vi "Readable.vi"(8 "error in (no error)":errorcluster, 9 "Channel Units":T1, 10 "Channel Names":T2, 11 "Readable in":refnum<class "Readable.lvclass">) -> (0 "error out":errorcluster, 3 "Readable out":refnum<class "Readable.lvclass">)   [LabVIEW 2017, in "Readable.lvclass"]
uses:
  Readable.lvclass
  Channel Names.ctl
  Channel Units.ctl
  Data Point.ctl
  Time.ctl
  X.ctl
  Readable.lvclass/Readable.ctl
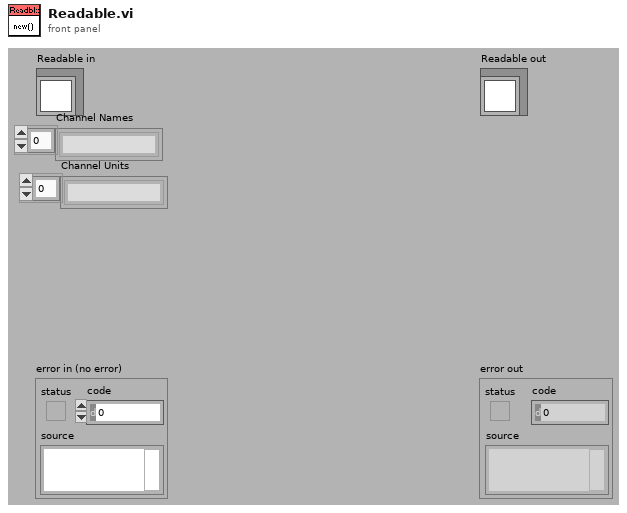
[diagram p1: front panel]
types:
  T1 = typedef "Readable.lvclass/Channel Units.ctl" = string[]
  T2 = typedef "Readable.lvclass/Channel Names.ctl" = string[]
  T3 = typedef "Readable.lvclass/Data Point.ctl" = cluster{"t":T4, "x":T5}
  T4 = typedef "Readable.lvclass/Time.ctl" = timestamp
  T5 = typedef "Readable.lvclass/X.ctl" = dbl
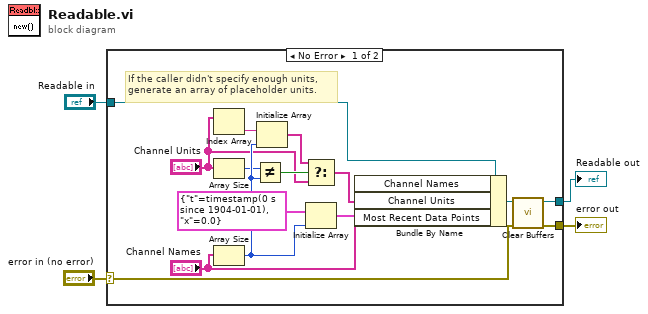
[diagram p0: block diagram]
diagram:
  n1 = case shown="No Error" "error in (no error)" {
    selector: "error in (no error)" -> [w6 w21]
    tunnel: [w5 w21] -> w3
    tunnel: [w7 w20] -> w1
    tunnel: "Readable in" -> [w19 w20]
    frame No Error {
      # "If the caller didn't specify enough units,\ngenerate an array of placeholder units."
      n2 = Index Array(array="Channel Units") -> (element=w9:string)  [unwired: 1 in]
      n3 = Array Size(array="Channel Units") -> (size(s)=w12:i32)
      n4 = Array Size(array="Channel Names") -> (size(s)=w13:i32)
      n5 = Not Equal?(x=w12, y=w13) -> (x != y?=w11:bool)
      n6 = Initialize Array(w9, w13) -> (w15:string[])
      n7 = Select(t=w15, s=w11, f="Channel Units") -> (s? t:f=w14:T1)
      n8 = Initialize Array(T3 {"t"=timestamp(0 s since 1904-01-01), "x"=0.0} ("Data Point"), w13) -> (w17:T3[])
      n9 = Bundle By Name(cluster=w19, "Channel Names"="Channel Names", "Channel Units"=w14, "Most Recent Data Points"=w17) -> (w18:refnum<class "Readable.lvclass">)
      n10 = call "Clear Buffers.vi"("error in (no error)"=w6, "Readable in"=w18) -> ("error out"=w5:errorcluster, "Readable out"=w7:refnum<class "Readable.lvclass">)  [unwired: 8 in]
    }
    frame Error {
    }
  }
  "error out" <- w3
  "Readable out" <- w1
